vi "_REP_FrontLabel.vi"(11 "label":string) -> (3 "String":string)   [LabVIEW 2014]
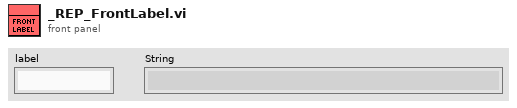
[diagram p1: front panel]
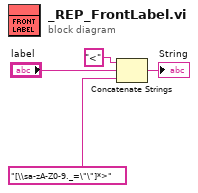
[diagram p0: block diagram]
diagram:
  n1 = Concatenate Strings("<" ("regular expression"), "label", "[\\sa-zA-Z0-9._=\"\"]*>" ("regular expression")) -> (→"String":string)
